vi "nana_4-ZN_O.vi"() -> ()   [LabVIEW 2015]
uses:
  <vilib>/MakerHub/LINX/Public/Peripherals/Digital/Digital Write N Chans.vi
  <vilib>/MakerHub/LINX/Public/Peripherals/Analog/Analog Read 1 Chan.vi
  <vilib>/MakerHub/LINX/Private/Local IO/LinxDigitalWrite.vi
  <vilib>/MakerHub/LINX/Public/Utilities/Check Channel.vi
  <vilib>/MakerHub/LINX/Public/Peripherals/Analog/Analog Read N Chans.vi
  <vilib>/MakerHub/LINX/Private/Local IO/LinxAnalogRead.vi
  <vilib>/MakerHub/LINX/Public/Utilities/Open Serial.vi
  <vilib>/MakerHub/LINX/Private/Utilties/Generate Error.vi
  <vilib>/MakerHub/LINX/LMH-LINX.lvlib
panel:
  in  "time post":u32
  in  "number of pulses":i32
  in  "low delay":u32
  in  "peak delay":u32
  out "Ref":dbl(graph)
  in  "LED":refnum<visa-resource-name>="N/A"
  out "3":dbl(graph)
  out "2":dbl(graph)
  out "4":dbl(graph)
  out "1":dbl(graph)
  out "pos":dbl
  in  "milliseconds to wait":u32
  in  "time pre":u32
  in  "Serial Port Analog":refnum<visa-resource-name>="N/A"
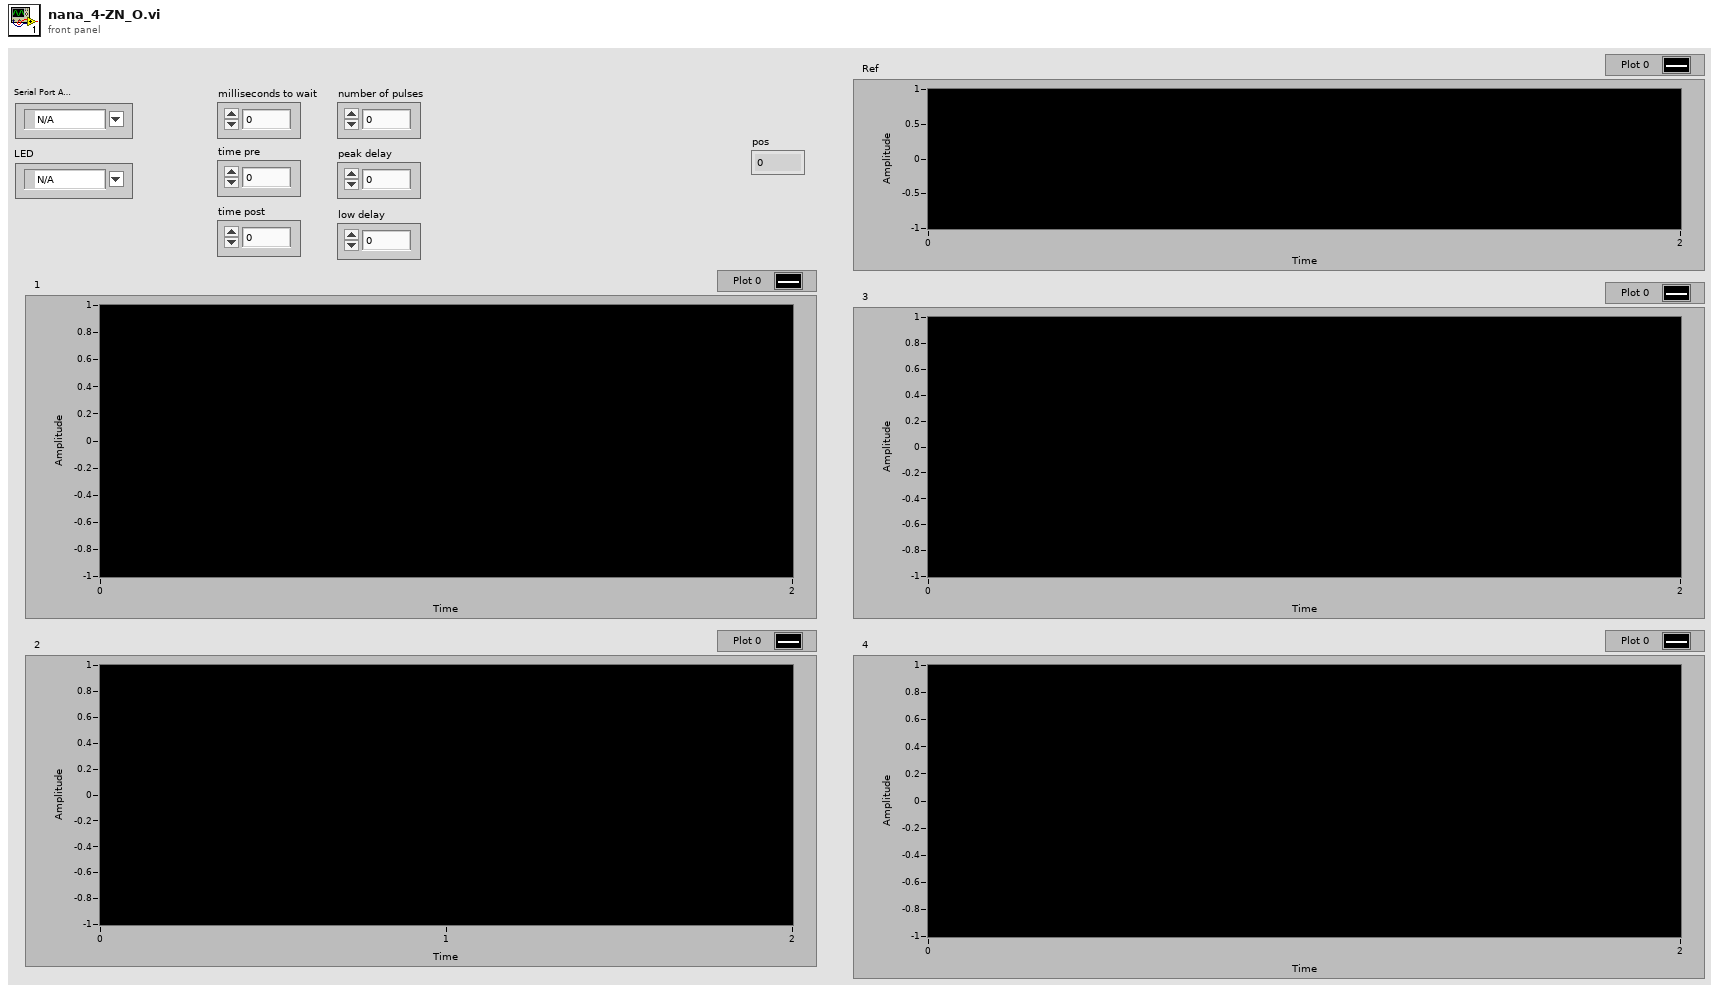
[diagram p1: front panel]
types:
  T1 = typedef "LMH-LINX.lvlib/LINX Ref.ctl" = cluster{"IO":T2, "Interface":T3, "LINX Device Config":T4}
  T2 = typedef "LMH-LINX.lvlib/Platform.ctl" = enum16{"Remote", "Local"}
  T3 = typedef "LMH-LINX.lvlib/Interface.ctl" = enum16{"Serial", "TCP"}
  T4 = typedef "LMH-LINX.lvlib/Device.lvlib/LINX Device Config.ctl" = cluster{"Interface":T3, "COM Port":refnum<visa-resource-name>, "TCP Configuration":T5, "Device Family":u8, "Device ID":u8, "Device Name":string, "TCP Ref":refnum<k5>, "Channels":T6}
  T5 = typedef "LMH-LINX.lvlib/Device.lvlib/TCP Config.ctl" = cluster{"IP Address":string, "Port":u16}
  T6 = typedef "LMH-LINX.lvlib/Channels.ctl" = cluster{"DI":u8[], "DO":u8[], "AI":u8[], "AO":u8[], "PWM":u8[], "QE":u8[], "UART":u8[], "I2C 2":u8[], "SPI":u8[], "CAN":u8[], "Servo":u8[], "AI Ref (V)":dbl, "AI Resolution (Bits)":u8, "AO Ref (V)":dbl, "AO Resolution (Bits)":u8}
  T7 = enum16{"open", "replace", "create", "open or create", "replace or create", "replace or create with confirmation"}
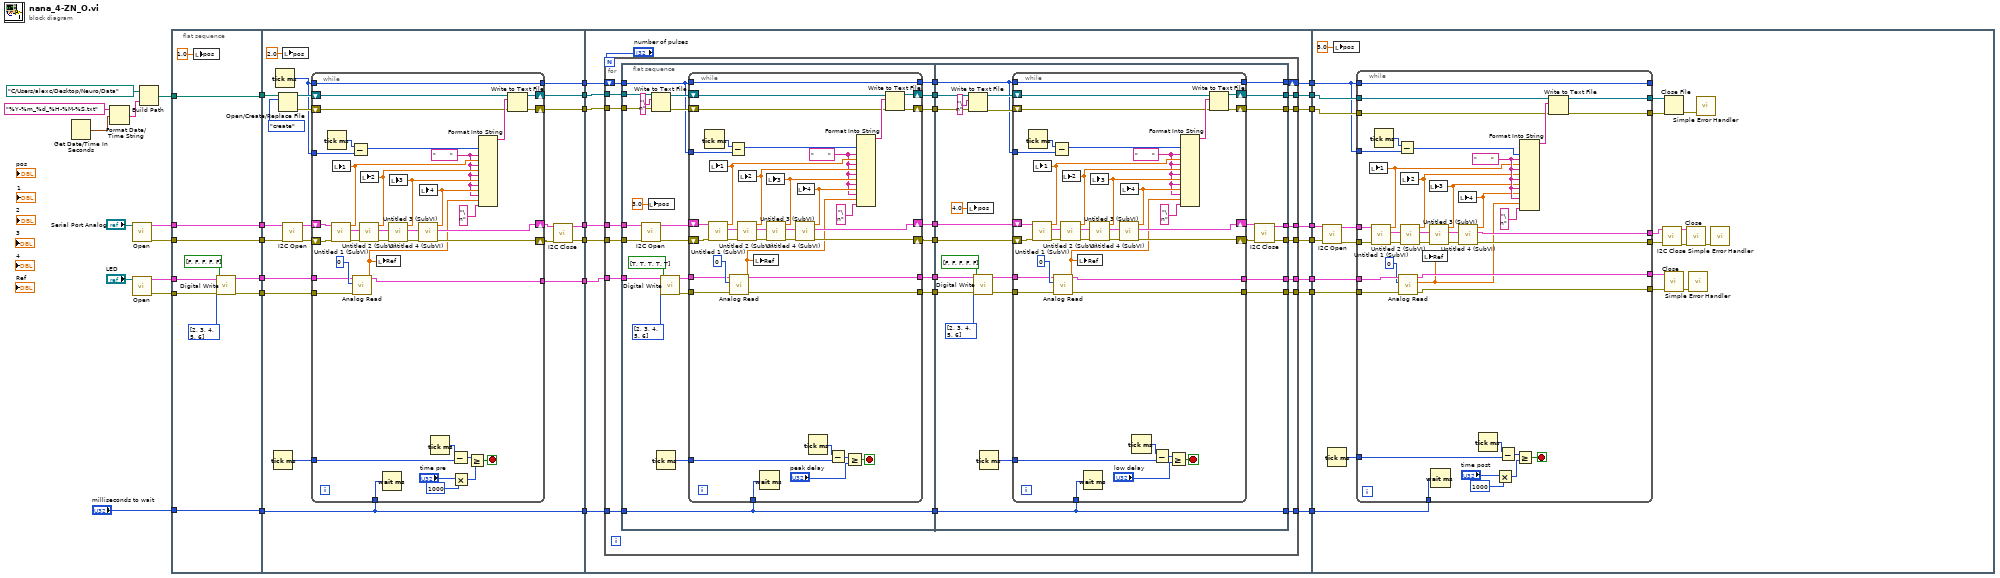
[diagram p0: block diagram]
diagram:
  n1 = Get Date/Time In Seconds() -> (seconds since 1Jan1904=w11:timestamp)
  n2 = Format Date/Time String(time format string (%c)="%Y-%m_%d_%H-%M-%S.txt", seconds (now)=w11) -> (date/time string=w13:string)  [unwired: 1 in]
  n3 = call-poly <vilib>:"Open.vi"("Serial Port"="Serial Port Analog") -> ("Error Out"=w17:errorcluster, "LINX Resource"=w18:T1)  [unwired: 8 in, 1 out]
  n4 = call-poly <vilib>:"Open.vi"("Serial Port"="LED") -> ("Error Out"=w8:errorcluster, "LINX Resource"=w9:T1)  [unwired: 8 in, 1 out]
  n5 = Build Path(base path=path "C:/Users/alexc/Desktop/Neuro/Data", name or relative path=w13) -> (appended path=w10:path)
  n6 = flat-sequence {
    tunnel: [w41] -> w33
    tunnel: [w40] -> w32
    tunnel: [w39] -> w29
    tunnel: [w34] -> w20
    tunnel: w18 -> [w41]
    tunnel: w17 -> [w40]
    tunnel: w10 -> [w39]
    tunnel: w9 -> [w38]
    tunnel: w8 -> [w37]
    tunnel: [w36] -> w7
    tunnel: [w35] -> w6
    tunnel: "milliseconds to wait" -> [w34]
    tunnel: w33 -> [w66]
    tunnel: w32 -> [w65]
    tunnel: [w64] -> w31
    tunnel: [w63] -> w30
    tunnel: w29 -> [w62]
    tunnel: [w58] -> w28
    tunnel: [w57] -> w27
    tunnel: [w55] -> w26
    tunnel: w20 -> [w53]
    tunnel: [w53] -> w19
    tunnel: w7 -> [w47]
    tunnel: w6 -> [w46]
    tunnel: [w45] -> w5
    tunnel: [w109] -> w25
    tunnel: [w108] -> w24
    tunnel: [w112] -> w23
    tunnel: [w111] -> w22
    tunnel: [w110] -> w21
    tunnel: w19 -> [w113]
    tunnel: w26 -> [w117]
    tunnel: w27 -> [w118]
    tunnel: w28 -> [w119]
    tunnel: w30 -> [w115]
    tunnel: w31 -> [w116]
    tunnel: w5 -> [w120]
    tunnel: [w107] -> w3
    tunnel: [w106] -> w2
    tunnel: [w105] -> w1
    tunnel: w21 -> [w282]
    tunnel: w22 -> [w283]
    tunnel: w23 -> [w269]
    tunnel: w24 -> [w287]
    tunnel: w25 -> [w291]
    tunnel: w3 -> [w286]
    tunnel: w2 -> [w273]
    tunnel: w1 -> [w272]
    frame #0 {
      n7 = local write "pos"(1.0 ("pos")) -> ()
      n8 = call-poly <vilib>:"Digital Write.vi"("Error In"=w37, "Values"=bool[] [FALSE, FALSE, FALSE, FALSE, FALSE], "DO Channels"=u8[] [2, 3, 4, 5, 6], "LINX Resource"=w38) -> ("Error Out"=w35:errorcluster, "LINX Resource"=w36:T1)  [unwired: 6 in]
    }
    frame #1 {
      n9 = Tick Count (ms)() -> (millisecond timer value=w54:u32)
      n10 = Tick Count (ms)() -> (millisecond timer value=w56:u32)
      n11 = Open/Create/Replace File(file path (use dialog)=w62, operation (0:open)=T7."create") -> (refnum out=w60:refnum<file>, error out=w59:errorcluster)  [unwired: 4 in, 1 out]
      n12 = local write "pos"(2.0 ("pos")) -> ()
      n13 = call <vilib>:"I2C Open.vi"("Error In"=w65, "LINX Resource"=w66) -> ("Error Out"=w51:errorcluster, "LINX Resource"=w52:T1)  [unwired: 8 in]
      n14 = while {
        tunnel: w56 -> [w97]
        shift-right: [w93] -> w58
        shift-left: w60 -> [w95]
        shift-right: [w92] -> w57
        shift-left: w59 -> [w94]
        tunnel: [w91] -> w55
        tunnel: w56 -> [w91]
        tunnel: w54 -> [w71]
        tunnel: w53 -> [w75]
        shift-right: [w88] -> w50
        shift-left: w52 -> [w90]
        shift-right: [w87] -> w49
        shift-left: w51 -> [w89]
        tunnel: w47 -> [w77]
        tunnel: w46 -> [w76]
        tunnel: [w74] -> w45
        stop <- w70 stop-if-true
        w81 = "       "
        n15 = Tick Count (ms)() -> (millisecond timer value=w98:u32)
        n16 = call "Untitled 1 (SubVI).vi"("error in (no error)"=w89, "LINX Resource in"=w90) -> ("error out"=w103:errorcluster, "LINX Resource out"=w104:T1, "Numeric"=w85:dbl)  [unwired: 7 in]
        n17 = local write "1"(w85) -> ()
        n18 = Subtract(x=w98, y=w97) -> (x-y=w82:u32)
        n19 = call-poly <vilib>:"Analog Read.vi"("Error In"=w76, "Analog Channel"=u8 0, "LINX Resource"=w77) -> ("Voltage"=w78:dbl, "LINX Resource"=w74:T1)  [unwired: 5 in, 2 out]
        n20 = call "Untitled 2 (SubVI).vi"("error in (no error)"=w103, "LINX Resource in"=w104) -> ("error out"=w102:errorcluster, "LINX Resource"=w101:T1, "Numeric"=w84:dbl)  [unwired: 7 in]
        n21 = local write "2"(w84) -> ()
        n22 = local write "Ref"(w78) -> ()
        n23 = Wait (ms)(milliseconds to wait=w75) -> ()  [unwired: 1 out]
        n24 = call "Untitled 3 (SubVI).vi"("error in (no error)"=w102, "LINX Resource in"=w101) -> ("error out"=w99:errorcluster, "LINX Resource out"=w100:T1, "Numeric"=w83:dbl)  [unwired: 7 in]
        n25 = local write "3"(w83) -> ()
        n26 = call "Untitled 4 (SubVI).vi"("error in (no error)"=w99, "LINX Resource in"=w100) -> ("error out"=w87:errorcluster, "LINX Resource"=w88:T1, "Numeric"=w86:dbl)  [unwired: 7 in]
        n27 = local write "4"(w86) -> ()
        n28 = Tick Count (ms)() -> (millisecond timer value=w72:u32)
        n29 = Subtract(x=w72, y=w71) -> (x-y=w73:u32)
        n30 = Multiply(x="time pre", y=u32 1000) -> (x*y=w69:u32)
        n31 = Greater Or Equal?(x=w73, y=w69) -> (x >= y?=w70:bool)
        n32 = Format Into String(w82, w81, w85, w81, w84, w81, w83, w81, w86, w81, w78, "\n") -> (resulting string=w96:string)  [unwired: 3 in, 1 out]
        n33 = Write to Text File(file (use dialog)=w95, text=w96, error in=w94) -> (refnum out=w93:refnum<file>, error out=w92:errorcluster)  [unwired: 1 in, 1 out]
      }
      n34 = call <vilib>:"I2C Close.vi"("Error In"=w49, "LINX Resource"=w50) -> ("Error Out"=w63:errorcluster, "LINX Resource"=w64:T1)  [unwired: 8 in]
    }
    frame #2 {
      n35 = for {
        N: "number of pulses" -> [_]
        tunnel: w120 -> [w143]
        tunnel: w119 -> [w142]
        tunnel: w118 -> [w141]
        shift-right: [w128] -> w112
        shift-left: w117 -> [w138]
        tunnel: w116 -> [w140]
        tunnel: w115 -> [w139]
        tunnel: w113 -> [w130]
        tunnel: [w127] -> w111
        tunnel: [w126] -> w110
        tunnel: [w125] -> w109
        tunnel: [w124] -> w108
        tunnel: [w123] -> w107
        tunnel: [w122] -> w106
        tunnel: [w121] -> w105
        n36 = flat-sequence {
          tunnel: w143 -> [w163]
          tunnel: w142 -> [w160]
          tunnel: w141 -> [w159]
          tunnel: w140 -> [w152]
          tunnel: w139 -> [w151]
          tunnel: w138 -> [w148]
          tunnel: [w167] -> w137
          tunnel: [w166] -> w136
          tunnel: [w162] -> w135
          tunnel: [w161] -> w134
          tunnel: [w156] -> w133
          tunnel: [w155] -> w132
          tunnel: [w147] -> w131
          tunnel: w130 -> [w144]
          tunnel: [w144] -> w129
          tunnel: w137 -> [w224]
          tunnel: w136 -> [w223]
          tunnel: w135 -> [w218]
          tunnel: w134 -> [w217]
          tunnel: w133 -> [w220]
          tunnel: w132 -> [w219]
          tunnel: w131 -> [w216]
          tunnel: w129 -> [w208]
          tunnel: [w213] -> w128
          tunnel: [w212] -> w127
          tunnel: [w211] -> w126
          tunnel: [w210] -> w125
          tunnel: [w209] -> w124
          tunnel: [w208] -> w123
          tunnel: [w207] -> w122
          tunnel: [w206] -> w121
          frame #0 {
            n37 = call <vilib>:"I2C Open.vi"("Error In"=w151, "LINX Resource"=w152) -> ("Error Out"=w149:errorcluster, "LINX Resource"=w150:T1)  [unwired: 8 in]
            n38 = local write "pos"(3.0 ("pos")) -> ()
            n39 = Write to Text File(file (use dialog)=w160, text="\n", error in=w159) -> (refnum out=w158:refnum<file>, error out=w157:errorcluster)  [unwired: 1 in, 1 out]
            n40 = Tick Count (ms)() -> (millisecond timer value=w145:u32)
            n41 = call-poly <vilib>:"Digital Write.vi"("Values"=bool[] [TRUE, TRUE, TRUE, TRUE, TRUE], "DO Channels"=u8[] [2, 3, 4, 5, 6], "LINX Resource"=w163) -> ("Error Out"=w154:errorcluster, "LINX Resource"=w153:T1)  [unwired: 7 in]
            n42 = while {
              tunnel: w148 -> [w198]
              shift-right: [w194] -> w162
              shift-left: w158 -> [w196]
              shift-right: [w193] -> w161
              shift-left: w157 -> [w195]
              tunnel: [w192] -> w147
              tunnel: w148 -> [w192]
              tunnel: w145 -> [w169]
              tunnel: w144 -> [w176]
              shift-right: [w189] -> w167
              shift-left: w150 -> [w191]
              shift-right: [w188] -> w166
              shift-left: w149 -> [w190]
              tunnel: w153 -> [w178]
              tunnel: w154 -> [w177]
              tunnel: [w175] -> w156
              tunnel: [w174] -> w155
              stop <- w171 stop-if-true
              w182 = "       "
              n43 = Tick Count (ms)() -> (millisecond timer value=w199:u32)
              n44 = call "Untitled 1 (SubVI).vi"("error in (no error)"=w190, "LINX Resource in"=w191) -> ("error out"=w204:errorcluster, "LINX Resource out"=w205:T1, "Numeric"=w186:dbl)  [unwired: 7 in]
              n45 = local write "1"(w186) -> ()
              n46 = Subtract(x=w199, y=w198) -> (x-y=w183:u32)
              n47 = call-poly <vilib>:"Analog Read.vi"("Error In"=w177, "Analog Channel"=u8 0, "LINX Resource"=w178) -> ("Error Out"=w174:errorcluster, "Voltage"=w179:dbl, "LINX Resource"=w175:T1)  [unwired: 5 in, 1 out]
              n48 = call "Untitled 2 (SubVI).vi"("error in (no error)"=w204, "LINX Resource in"=w205) -> ("error out"=w203:errorcluster, "LINX Resource"=w202:T1, "Numeric"=w185:dbl)  [unwired: 7 in]
              n49 = local write "2"(w185) -> ()
              n50 = local write "Ref"(w179) -> ()
              n51 = Wait (ms)(milliseconds to wait=w176) -> ()  [unwired: 1 out]
              n52 = call "Untitled 3 (SubVI).vi"("error in (no error)"=w203, "LINX Resource in"=w202) -> ("error out"=w200:errorcluster, "LINX Resource out"=w201:T1, "Numeric"=w184:dbl)  [unwired: 7 in]
              n53 = local write "3"(w184) -> ()
              n54 = call "Untitled 4 (SubVI).vi"("error in (no error)"=w200, "LINX Resource in"=w201) -> ("error out"=w188:errorcluster, "LINX Resource"=w189:T1, "Numeric"=w187:dbl)  [unwired: 7 in]
              n55 = local write "4"(w187) -> ()
              n56 = Tick Count (ms)() -> (millisecond timer value=w172:u32)
              n57 = Subtract(x=w172, y=w169) -> (x-y=w173:u32)
              n58 = Greater Or Equal?(x=w173, y="peak delay") -> (x >= y?=w171:bool)
              n59 = Format Into String(w183, w182, w186, w182, w185, w182, w184, w182, w187, w182, w179, "\n") -> (resulting string=w197:string)  [unwired: 3 in, 1 out]
              n60 = Write to Text File(file (use dialog)=w196, text=w197, error in=w195) -> (refnum out=w194:refnum<file>, error out=w193:errorcluster)  [unwired: 1 in, 1 out]
            }
          }
          frame #1 {
            n61 = local write "pos"(4.0 ("pos")) -> ()
            n62 = Write to Text File(file (use dialog)=w218, text="\n", error in=w217) -> (refnum out=w226:refnum<file>, error out=w227:errorcluster)  [unwired: 1 in, 1 out]
            n63 = call-poly <vilib>:"Digital Write.vi"("Error In"=w219, "Values"=bool[] [FALSE, FALSE, FALSE, FALSE, FALSE], "DO Channels"=u8[] [2, 3, 4, 5, 6], "LINX Resource"=w220) -> ("Error Out"=w231:errorcluster, "LINX Resource"=w230:T1)  [unwired: 6 in]
            n64 = Tick Count (ms)() -> (millisecond timer value=w214:u32)
            n65 = while {
              tunnel: w216 -> [w261]
              shift-right: [w257] -> w212
              shift-left: w226 -> [w259]
              shift-right: [w256] -> w211
              shift-left: w227 -> [w258]
              tunnel: [w255] -> w213
              tunnel: w216 -> [w255]
              tunnel: w214 -> [w234]
              tunnel: w208 -> [w239]
              shift-right: [w252] -> w222
              shift-left: w224 -> [w254]
              shift-right: [w251] -> w221
              shift-left: w223 -> [w253]
              tunnel: w230 -> [w241]
              tunnel: w231 -> [w240]
              tunnel: [w238] -> w207
              tunnel: [w237] -> w206
              stop <- w232 stop-if-true
              w245 = "       "
              n66 = Tick Count (ms)() -> (millisecond timer value=w262:u32)
              n67 = call "Untitled 1 (SubVI).vi"("error in (no error)"=w253, "LINX Resource in"=w254) -> ("error out"=w267:errorcluster, "LINX Resource out"=w268:T1, "Numeric"=w249:dbl)  [unwired: 7 in]
              n68 = local write "1"(w249) -> ()
              n69 = Subtract(x=w262, y=w261) -> (x-y=w246:u32)
              n70 = call-poly <vilib>:"Analog Read.vi"("Error In"=w240, "Analog Channel"=u8 0, "LINX Resource"=w241) -> ("Error Out"=w237:errorcluster, "Voltage"=w242:dbl, "LINX Resource"=w238:T1)  [unwired: 5 in, 1 out]
              n71 = call "Untitled 2 (SubVI).vi"("error in (no error)"=w267, "LINX Resource in"=w268) -> ("error out"=w266:errorcluster, "LINX Resource"=w265:T1, "Numeric"=w248:dbl)  [unwired: 7 in]
              n72 = local write "2"(w248) -> ()
              n73 = local write "Ref"(w242) -> ()
              n74 = Wait (ms)(milliseconds to wait=w239) -> ()  [unwired: 1 out]
              n75 = call "Untitled 3 (SubVI).vi"("error in (no error)"=w266, "LINX Resource in"=w265) -> ("error out"=w263:errorcluster, "LINX Resource out"=w264:T1, "Numeric"=w247:dbl)  [unwired: 7 in]
              n76 = local write "3"(w247) -> ()
              n77 = call "Untitled 4 (SubVI).vi"("error in (no error)"=w263, "LINX Resource in"=w264) -> ("error out"=w251:errorcluster, "LINX Resource"=w252:T1, "Numeric"=w250:dbl)  [unwired: 7 in]
              n78 = local write "4"(w250) -> ()
              n79 = Tick Count (ms)() -> (millisecond timer value=w235:u32)
              n80 = Subtract(x=w235, y=w234) -> (x-y=w236:u32)
              n81 = Greater Or Equal?(x=w236, y="low delay") -> (x >= y?=w232:bool)
              n82 = Format Into String(w246, w245, w249, w245, w248, w245, w247, w245, w250, w245, w242, "\n") -> (resulting string=w260:string)  [unwired: 3 in, 1 out]
              n83 = Write to Text File(file (use dialog)=w259, text=w260, error in=w258) -> (refnum out=w257:refnum<file>, error out=w256:errorcluster)  [unwired: 1 in, 1 out]
            }
            n84 = call <vilib>:"I2C Close.vi"("Error In"=w221, "LINX Resource"=w222) -> ("Error Out"=w209:errorcluster, "LINX Resource"=w210:T1)  [unwired: 8 in]
          }
        }
      }
    }
    frame #3 {
      n85 = call <vilib>:"I2C Open.vi"("Error In"=w287, "LINX Resource"=w291) -> ("Error Out"=w284:errorcluster, "LINX Resource"=w285:T1)  [unwired: 8 in]
      n86 = Tick Count (ms)() -> (millisecond timer value=w281:u32)
      n87 = local write "pos"(5.0 ("pos")) -> ()
      n88 = while {
        tunnel: w286 -> [w324]
        tunnel: w285 -> [w323]
        tunnel: w284 -> [w322]
        tunnel: [w316] -> _
        tunnel: w269 -> [w316]
        tunnel: w283 -> [w315]
        tunnel: w282 -> [w314]
        tunnel: w281 -> [w295]
        tunnel: [w313] -> w280
        tunnel: [w312] -> w279
        tunnel: [w311] -> w276
        tunnel: [w310] -> w275
        tunnel: w273 -> [w309]
        tunnel: w272 -> [w308]
        tunnel: [w307] -> w271
        tunnel: [w306] -> w270
        tunnel: w269 -> [w304]
        stop <- w296 stop-if-true
        w326 = "       "
        n89 = call "Untitled 1 (SubVI).vi"("error in (no error)"=w322, "LINX Resource in"=w323) -> ("error out"=w321:errorcluster, "LINX Resource out"=w330:T1, "Numeric"=w318:dbl)  [unwired: 7 in]
        n90 = local write "1"(w318) -> ()
        n91 = Tick Count (ms)() -> (millisecond timer value=w317:u32)
        n92 = Subtract(x=w317, y=w304) -> (x-y=w303:u32)
        n93 = call-poly <vilib>:"Analog Read.vi"("Error In"=w308, "Analog Channel"=u8 0, "LINX Resource"=w309) -> ("Error Out"=w306:errorcluster, "Voltage"=w302:dbl, "LINX Resource"=w307:T1)  [unwired: 5 in, 1 out]
        n94 = call "Untitled 2 (SubVI).vi"("error in (no error)"=w321, "LINX Resource in"=w330) -> ("error out"=w320:errorcluster, "LINX Resource"=w329:T1, "Numeric"=w301:dbl)  [unwired: 7 in]
        n95 = local write "2"(w301) -> ()
        n96 = local write "Ref"(w302) -> ()
        n97 = call "Untitled 3 (SubVI).vi"("error in (no error)"=w320, "LINX Resource in"=w329) -> ("error out"=w319:errorcluster, "LINX Resource out"=w328:T1, "Numeric"=w300:dbl)  [unwired: 7 in]
        n98 = local write "3"(w300) -> ()
        n99 = Wait (ms)(milliseconds to wait=w324) -> ()  [unwired: 1 out]
        n100 = call "Untitled 4 (SubVI).vi"("error in (no error)"=w319, "LINX Resource in"=w328) -> ("error out"=w310:errorcluster, "LINX Resource"=w311:T1, "Numeric"=w299:dbl)  [unwired: 7 in]
        n101 = local write "4"(w299) -> ()
        n102 = Tick Count (ms)() -> (millisecond timer value=w297:u32)
        n103 = Multiply(x="time post", y=u32 1000) -> (x*y=w294:u32)
        n104 = Subtract(x=w297, y=w295) -> (x-y=w298:u32)
        n105 = Greater Or Equal?(x=w298, y=w294) -> (x >= y?=w296:bool)
        n106 = Format Into String(w303, w326, w318, w326, w301, w326, w300, w326, w299, w326, w302, "\n") -> (resulting string=w327:string)  [unwired: 3 in, 1 out]
        n107 = Write to Text File(file (use dialog)=w315, text=w327, error in=w314) -> (refnum out=w313:refnum<file>, error out=w312:errorcluster)  [unwired: 1 in, 1 out]
      }
      n108 = call <vilib>:"I2C Close.vi"("Error In"=w275, "LINX Resource"=w276) -> ("Error Out"=w277:errorcluster, "LINX Resource"=w278:T1)  [unwired: 8 in]
      n109 = Close File(refnum=w280, error in=w279) -> (error out=w290:errorcluster)  [unwired: 1 out]
      n110 = call <vilib>:"Close.vi"("Error In"=w270, "LINX Resource"=w271) -> ("Error Out"=w274:errorcluster)  [unwired: 9 in]
      n111 = call <vilib>:"Close.vi"("Error In"=w277, "LINX Resource"=w278) -> ("Error Out"=w289:errorcluster)  [unwired: 9 in]
      n112 = call <vilib>:"Simple Error Handler.vi"("error in (no error)"=w274) -> ()  [unwired: 4 in, 5 out]
      n113 = call <vilib>:"Simple Error Handler.vi"("error in (no error)"=w290) -> ()  [unwired: 4 in, 5 out]
      n114 = call <vilib>:"Simple Error Handler.vi"("error in (no error)"=w289) -> ()  [unwired: 4 in, 5 out]
    }
  }
